vi "TEOAEs_Cecilia_Casarini.vi"() -> ()   [LabVIEW 2015]
uses:
  <vilib>/Utility/error.llb/DialogType.ctl
  <vilib>/DAQmx/write.llb/DAQmx Write (Analog 1D DBL 1Chan NSamp).vi
  <vilib>/DAQmx/read.llb/DAQmx Read (Analog Wfm 1Chan NSamp).vi
  <vilib>/addons/_NISVFA/_Baseband FFT/SVPO Power Spectrum (1 Ch DBL Array).vi
  <vilib>/addons/_NISVFA/_Baseband FFT/subVIs/svfa_Convert to One-Sided Power Spectrum.vi
  <vilib>/Analysis/2dsp.llb/Power Spectrum.vi
  <vilib>/Analysis/2dsp.llb/Power Spectrum (DBL).vi
  <vilib>/addons/_NISVFA/_Shared subVIs/Windowing/svfa_Scaled Time Domain Window (Array).vi
  <vilib>/Analysis/4window.llb/Force Window.vi
  <vilib>/Analysis/4window.llb/Force Window (DBL).vi
  <vilib>/Analysis/4window.llb/Exponential Window.vi
  <vilib>/Analysis/4window.llb/Exponential Window (DBL).vi
  <vilib>/DAQmx/create/channels.llb/DAQmx Create Channel (AI-Voltage-Basic).vi
  <vilib>/DAQmx/create/channels.llb/DAQmx Create Channel (AO-Voltage-Basic).vi
  <vilib>/DAQmx/configure/timing.llb/DAQmx Timing (Sample Clock).vi
  <vilib>/DAQmx/configure/trigger.llb/DAQmx Start Trigger (Digital Edge).vi
  <vilib>/DAQmx/miscellaneous.llb/DAQmx Fill In Error Info.vi
  <vilib>/addons/_NISVFA/_Spectrum Processing/subVIs/svfa_Spectrum Info Window to windowTd Type Def.vi
  <vilib>/Analysis/0measdsp.llb/Scaled Time Domain Window.vi
  <vilib>/Analysis/0measdsp.llb/Scaled Time Domain Window (DBL).vi
  <vilib>/Utility/error.llb/Error Cluster From Error Code.vi
  <vilib>/Analysis/NI_AALBase.lvlib
panel:
  in  "f2":dbl=0.5 format="%0.2f"
  in  "f1":dbl format="%0.2f"
  out "Non-aligned output/input waveforms":waveform(dbl)(graph)
  in  "Number of extra samples \nto READ from ADC":i32=200
  out "Input spectrum":cluster{"f0":dbl, "df":dbl, "magnitude":dbl[]}(graph)
  out "number of samples \nwritten per channel":u32
  in  "sampling info":cluster{"Fs":dbl, "samples in waveform":dbl}={"Fs"=204800.0, "samples in waveform"=1024.0} {"Fs" format="%.2p"}
  out "buffer size":i32
  in  "minimum value":dbl=-5.0 caption="Output Minimum Value" format="%0.2f"
  in  "maximum value":dbl=5.0 caption="Output Maximum Value" format="%0.2f"
  in  "physical channels":tag="PXI1Slot5/ao0" caption="Output Physical Channels"
  in  "Maximum Value":dbl=5.0 caption="Input Maximum Value" format="%0.2f"
  in  "Minimum Value":dbl=-5.0 caption="Input Minimum Value" format="%0.2f"
  in  "Physical Channel":tag="PXI1Slot5/ai0" caption="Input Physical Channel"
  out "Output waveform (samples)":dbl[](graph)
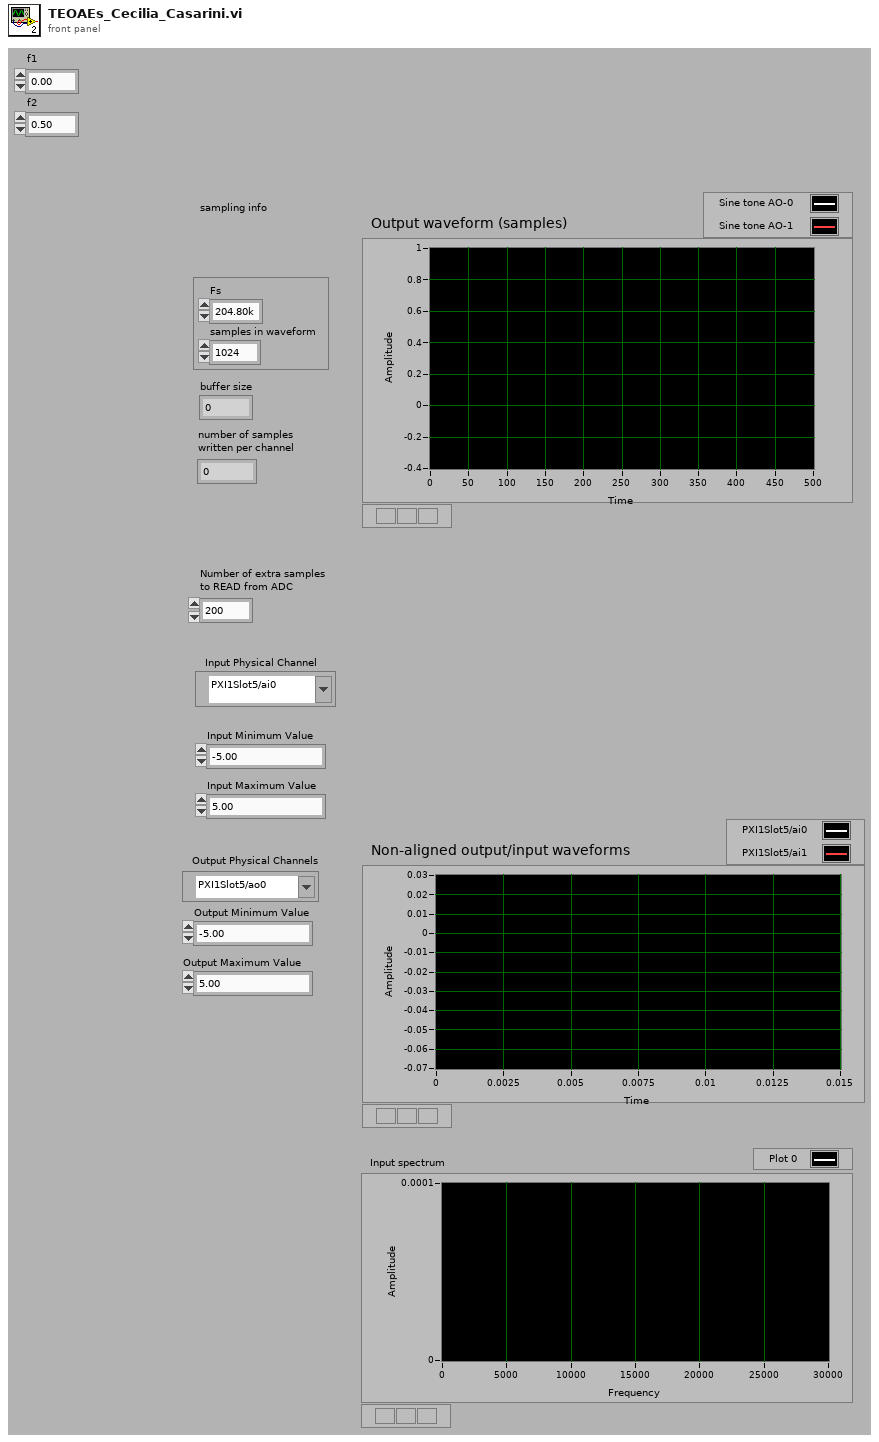
[diagram p1: front panel]
types:
  T1 = typedef "DialogType.ctl" = u16
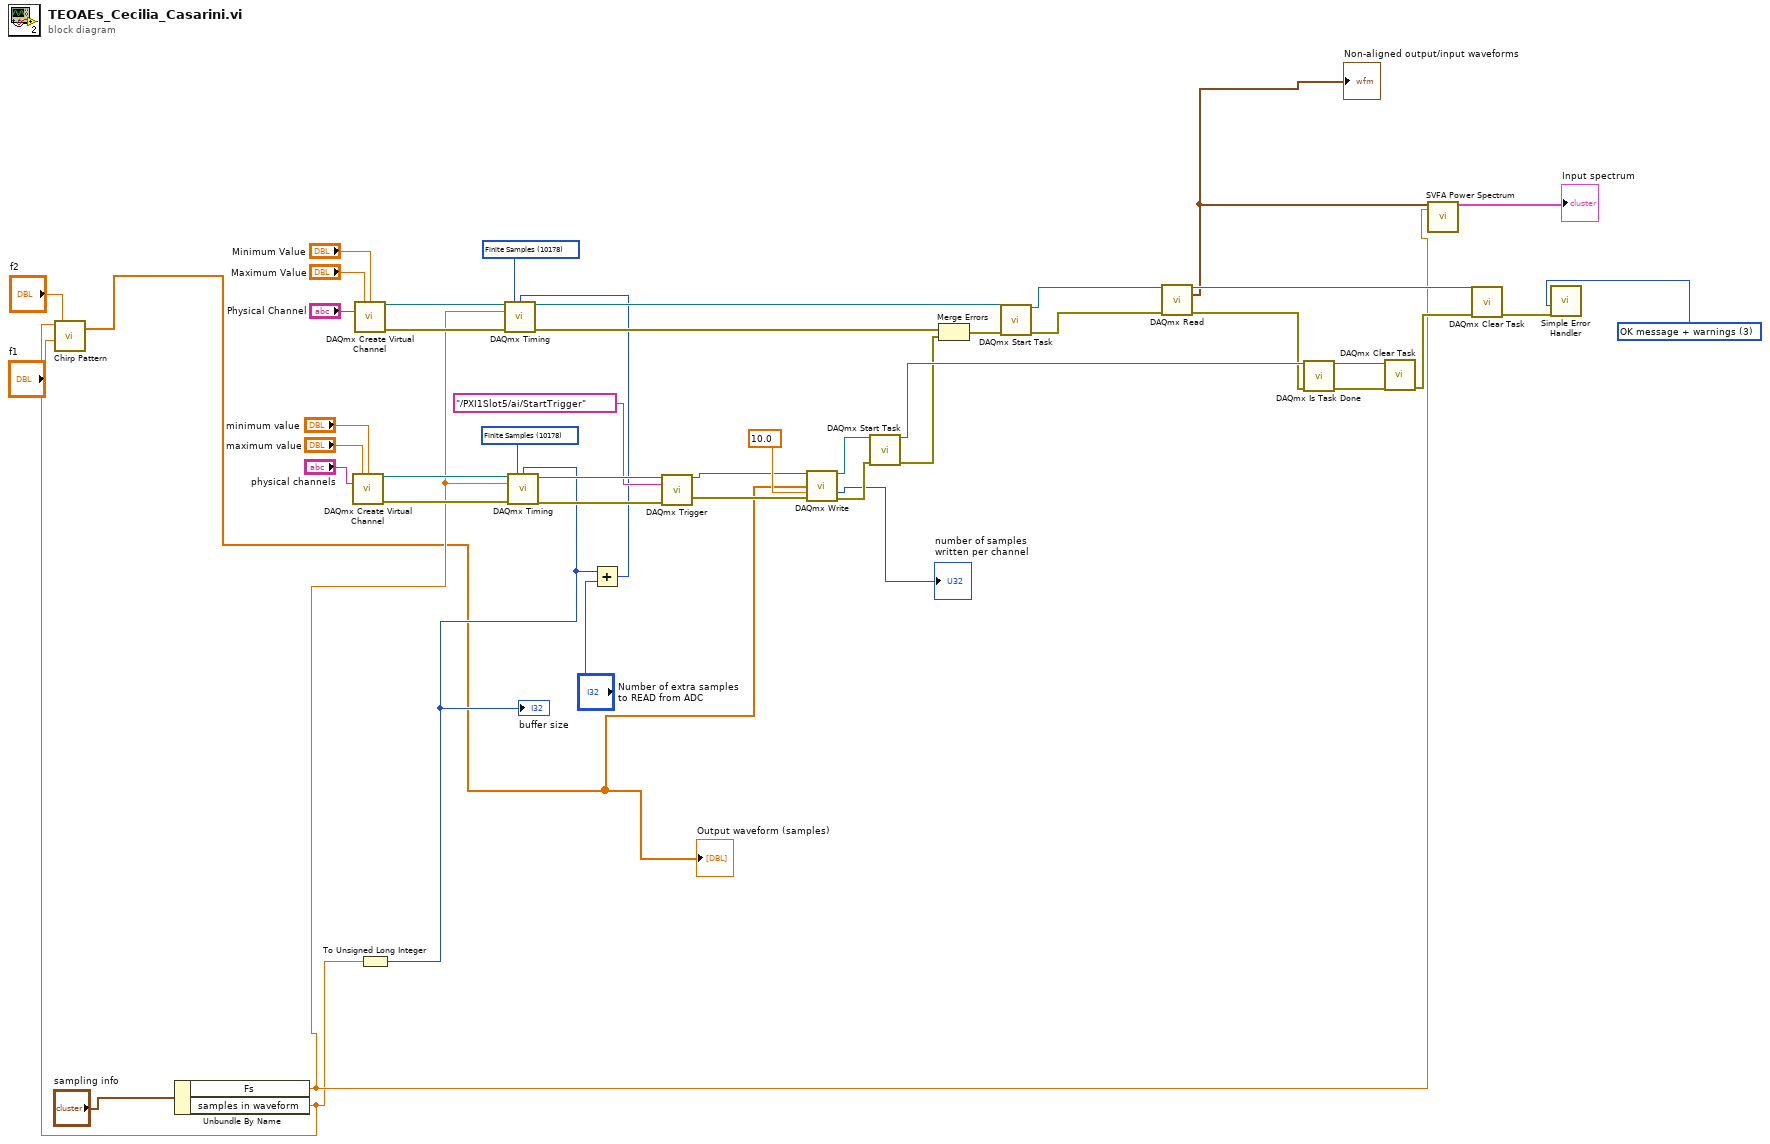
[diagram p0: block diagram]
diagram:
  w19 = T1 3 items=["no dialog", "OK message", "continue or stop message", "OK message + warnings", "continue/stop + warnings"] ("type of dialog (OK msg:1)")
  w39 = 10178 items=["Finite Samples"=10178, "Continuous Samples"=10123] ("sample mode")
  w44 = 10178 items=["Finite Samples"=10178, "Continuous Samples"=10123] ("sample mode")
  n1 = Unbundle By Name("sampling info") -> ("Fs"=w8:dbl, "samples in waveform"=w4:dbl)
  n2 = call <vilib>:"Chirp Pattern.vi"("f2"="f2", "f1"="f1", "samples"=w4) -> ("Chirp Pattern"=w3:dbl[])  [unwired: 1 in, 1 out]
  "Output waveform (samples)" <- w3
  n3 = call-poly <vilib>:"DAQmx Create Virtual Channel.vi"("maximum value"="maximum value", "minimum value"="minimum value", "physical channels"="physical channels") -> ("task out"=w38:refnum<k21>, "error out"=w37:errorcluster)  [unwired: 11 in]
  n4 = call-poly <vilib>:"DAQmx Create Virtual Channel.vi"("maximum value"="Maximum Value", "minimum value"="Minimum Value", "physical channels"="Physical Channel") -> ("task out"=w42:refnum<k21>, "error out"=w43:errorcluster)  [unwired: 11 in]
  n5 = To Unsigned Long Integer(number=w4) -> (unsigned 32bit integer=w7:u32)
  "buffer size" <- w7
  n6 = call-poly <vilib>:"DAQmx Timing.vi"("task/channels in"=w38, "sample mode"=w39, "samples per channel"=w7, "rate"=w8, "error in"=w37) -> ("task out"=w32:refnum<k21>, "error out"=w33:errorcluster)  [unwired: 9 in]
  n7 = Add(x=w7, y="Number of extra samples \nto READ from ADC") -> (x+y=w13:u32)
  n8 = call-poly <vilib>:"DAQmx Timing.vi"("task/channels in"=w42, "sample mode"=w44, "samples per channel"=w13, "rate"=w8, "error in"=w43) -> ("task out"=w16:refnum<k21>, "error out"=w17:errorcluster)  [unwired: 9 in]
  n9 = call-poly <vilib>:"DAQmx Trigger.vi"("task/channels in"=w32, "source"=tag "/PXI1Slot5/ai/StartTrigger", "error in"=w33) -> ("task out"=w27:refnum<k21>, "error out"=w28:errorcluster)  [unwired: 11 in]
  n10 = call-poly <vilib>:"DAQmx Write.vi"("task/channels in"=w27, "data"=w3, "timeout"=10.0 ("Wirite Timeout"), "error in"=w28) -> ("task out"=w30:refnum<k21>, "number of samples written per channel"=→"number of samples \nwritten per channel":u32, "error out"=w29:errorcluster)  [unwired: 9 in]
  n11 = call <vilib>:"DAQmx Start Task.vi"("task/channels in"=w30, "error in"=w29) -> ("task out"=w34:refnum<k21>, "error out"=w26:errorcluster)  [unwired: 12 in]
  n12 = Merge Errors(w17, w26) -> (w25:errorcluster)
  n13 = call <vilib>:"DAQmx Start Task.vi"("task/channels in"=w16, "error in"=w25) -> ("task out"=w35:refnum<k21>, "error out"=w36:errorcluster)  [unwired: 12 in]
  n14 = call-poly <vilib>:"DAQmx Read.vi"("task/channels in"=w35, "error in"=w36) -> ("task out"=w21:refnum<k21>, "data"=w5:waveform(dbl), "error out"=w12:errorcluster)  [unwired: 11 in]
  "Non-aligned output/input waveforms" <- w5
  n15 = call <vilib>:"DAQmx Is Task Done.vi"("task/channels in"=w34, "error in"=w12) -> ("task out"=w22:refnum<k21>, "error out"=w20:errorcluster)  [unwired: 11 in, 1 out]
  n16 = call <vilib>:"DAQmx Clear Task.vi"("task in"=w22, "error in"=w20) -> ("error out"=w11:errorcluster)  [unwired: 13 in]
  n17 = call-poly <vilib>:"SVFA Power Spectrum.vi"("scaled signal [EU]"=w5, "sampling rate [Hz]"=w8) -> ("power spectrum [EU^2 rms]"=→"Input spectrum":cluster{"f0":dbl, "df":dbl, "magnitude":dbl[]})  [unwired: 15 in, 2 out]
  n18 = call <vilib>:"DAQmx Clear Task.vi"("task in"=w21, "error in"=w11) -> ("error out"=w10:errorcluster)  [unwired: 13 in]
  n19 = call <vilib>:"Simple Error Handler.vi"("type of dialog (OK msg:1)"=w19, "error in (no error)"=w10) -> ()  [unwired: 3 in, 5 out]
